vi "chkArgCompToPar.vi"(8 "error in":errorcluster, 9 "argSN":i32, 10 "arg":string, 11 "par":string) -> (0 "error out":errorcluster, 3 "judgement":string)   [LabVIEW 2010]
panel:
  out "Enum":T1(ring)=enum."float"
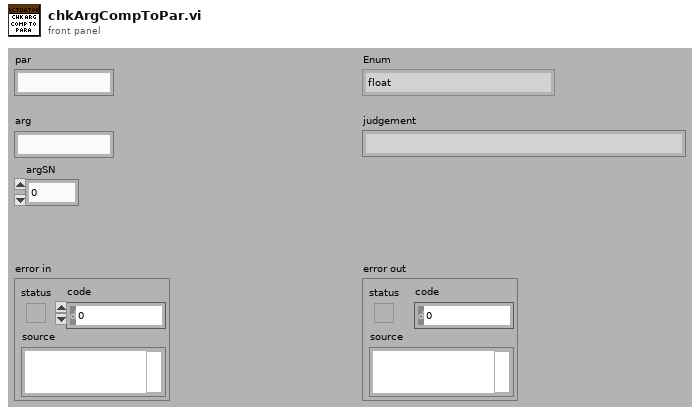
[diagram p1: front panel]
types:
  T1 = enum16{"char[]", "float", "double", "char", "int", "long", "dword", "qword", "enum"}
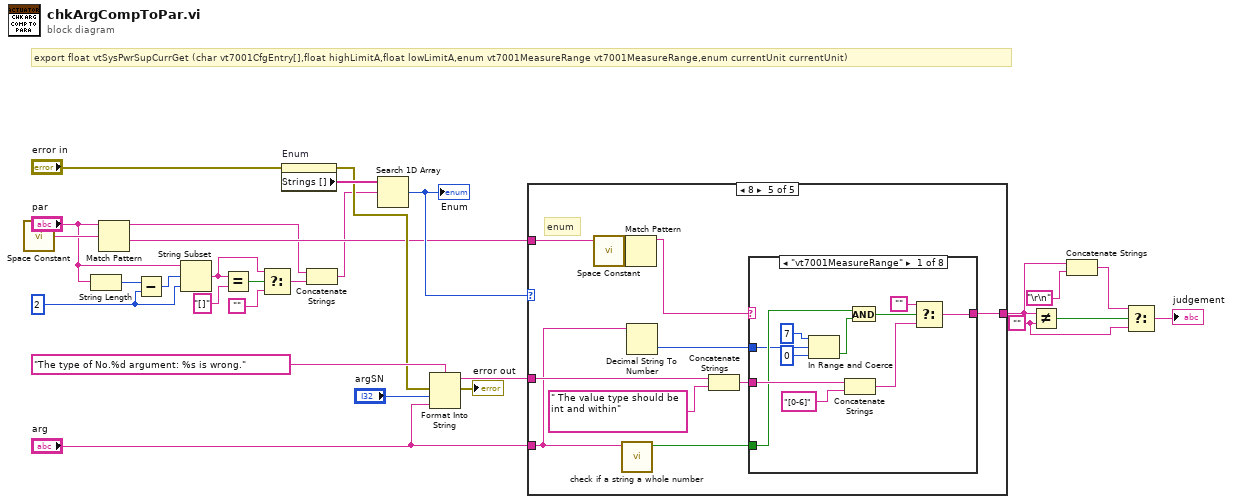
[diagram p0: block diagram]
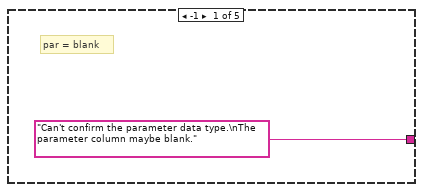
[diagram p2: hidden frame]
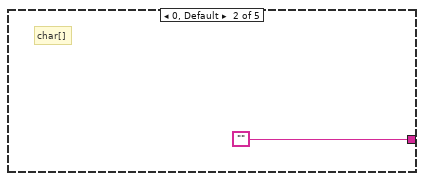
[diagram p3: hidden frame]
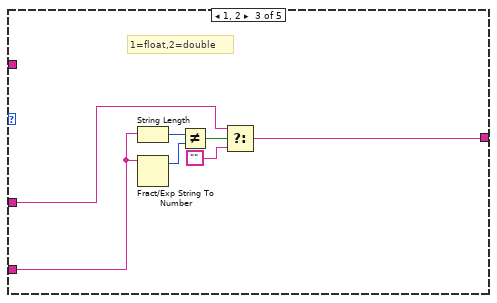
[diagram p4: hidden frame]
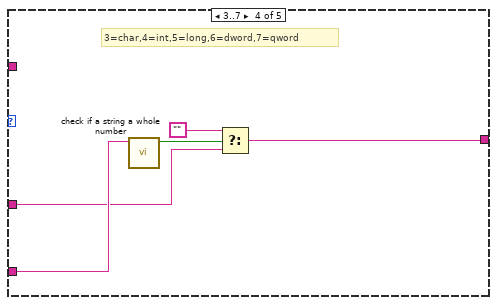
[diagram p5: hidden frame]
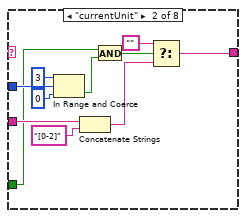
[diagram p6: hidden frame]
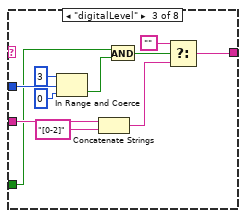
[diagram p7: hidden frame]
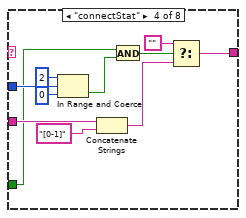
[diagram p8: hidden frame]
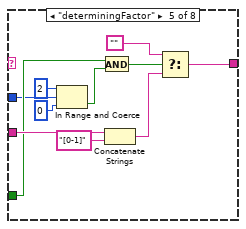
[diagram p9: hidden frame]
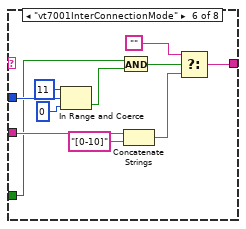
[diagram p10: hidden frame]
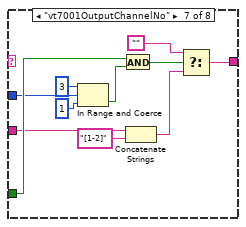
[diagram p11: hidden frame]
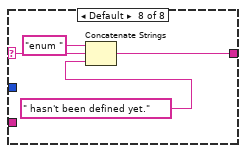
[diagram p12: hidden frame]
diagram:
  w2 = ""
  w14 = 2 ("y")
  # "export float vtSysPwrSupCurrGet (char vt7001CfgEntry[],float highLimitA,float lowLimitA,enum vt7001MeasureRange vt7001MeasureRange,enum currentUnit currentUnit)"
  n1 = call <vilib>:"Space Constant.vi"() -> ("String"=w28:string)
  n2 = String Length(string="par") -> (length=w17:i32)
  n3 = Match Pattern(string="par", regular expression=w28) -> (before substring=w8:string, after substring=w22:string)  [unwired: 1 in, 2 out]
  n4 = Subtract(x=w17, y=w14) -> (x-y=w15:i32)
  n5 = String Subset(string="par", offset (0)=w15, length (rest)=w14) -> (substring=w11:string)
  n6 = Equal?(x=w11, y="[]" ("String")) -> (x = y?=w12:bool)
  n7 = Select(t=w11, s=w12, f="") -> (s? t:f=w9:string)
  n8 = property on="Enum" class="Enum (strict)"(error in="error in") -> (error out=w24:errorcluster, "Strings []"=w27:string[])  [unwired: 1 in, 1 out]
  n9 = Concatenate Strings(w8, w9) -> (w7:string)
  n10 = Search 1D Array(1D array=w27, element=w7) -> (index of element=w26:i32)  [unwired: 1 in]
  "Enum" <- w26
  n11 = Format Into String(format string="The type of No.%d argument: %s is wrong.", error in=w24, "argSN", "arg") -> (resulting string=w23:string, error out=→"error out":errorcluster)  [unwired: 1 in]
  n12 = case shown="8" w26 {
    tunnel: "arg" -> [_ _ w35 w41 w45]
    tunnel: w23 -> [_ _ w31 w38 w47]
    tunnel: ["Can't confirm the parameter data type.\nThe parameter column maybe blank." "" w32 w42 w49] -> w4
    tunnel: w22 -> [_ _ _ _ w52]
    frame -1 {
      # "par = blank"
    }
    frame 0, Default {
      # "char[]"
    }
    frame 1, 2 {
      # "1=float,2=double"
      n13 = String Length(string=w35) -> (length=w37:i32)
      n14 = Fract/Exp String To Number(string=w35) -> (offset past number=w36:i32)  [unwired: 3 in, 1 out]
      n15 = Not Equal?(x=w37, y=w36) -> (x != y?=w34:bool)
      n16 = Select(t=w31, s=w34, f="") -> (s? t:f=w32:string)
    }
    frame 3..7 {
      # "3=char,4=int,5=long,6=dword,7=qword"
      n17 = call "check if a string a whole number.vi"("input string"=w41) -> ("is a whole number?"=w40:bool)  [unwired: 10 in]
      n18 = Select(t="", s=w40, f=w38) -> (s? t:f=w42:string)
    }
    frame 8 {
      # "enum"
      n19 = call <vilib>:"Space Constant.vi"() -> ("String"=w51:string)
      n20 = call "check if a string a whole number.vi"("input string"=w45) -> ("is a whole number?"=w48:bool)  [unwired: 10 in]
      n21 = Match Pattern(string=w52, regular expression=w51) -> (before substring=w50:string)  [unwired: 1 in, 3 out]
      n22 = Decimal String To Number(string=w45) -> (number=w44:i32)  [unwired: 2 in, 1 out]
      n23 = Concatenate Strings(w47, " The value type should be int and within" ("string")) -> (w46:string)
      n24 = case shown="\"vt7001MeasureRange\"" w50 {
        selector: w50 -> [_ _ _ _ _ _ _ w133]
        tunnel: w46 -> [w56 w67 w78 w89 w100 w110 w120 _]
        tunnel: [w55 w66 w77 w88 w101 w108 w119 w131] -> w49
        tunnel: w48 -> [w54 w64 w75 w86 w98 w109 w122 _]
        tunnel: w44 -> [w53 w65 w76 w87 w97 w111 w121 _]
        frame "vt7001MeasureRange" {
          n25 = In Range and Coerce(upper limit=7, x=w53, lower limit=0) -> (In Range?=w61:bool)  [unwired: 1 out]
          n26 = Concatenate Strings(w56, "[0-6]" ("string")) -> (w58:string)
          n27 = And(x=w54, y=w61) -> (x .and. y?=w60:bool)
          n28 = Select(t="", s=w60, f=w58) -> (s? t:f=w55:string)
        }
        frame "currentUnit" {
          n29 = In Range and Coerce(upper limit=3, x=w65, lower limit=0) -> (In Range?=w72:bool)  [unwired: 1 out]
          n30 = Concatenate Strings(w67, "[0-2]" ("string")) -> (w69:string)
          n31 = And(x=w64, y=w72) -> (x .and. y?=w71:bool)
          n32 = Select(t="", s=w71, f=w69) -> (s? t:f=w66:string)
        }
        frame "digitalLevel" {
          n33 = In Range and Coerce(upper limit=3, x=w76, lower limit=0) -> (In Range?=w83:bool)  [unwired: 1 out]
          n34 = Concatenate Strings(w78, "[0-2]" ("string")) -> (w80:string)
          n35 = And(x=w75, y=w83) -> (x .and. y?=w82:bool)
          n36 = Select(t="", s=w82, f=w80) -> (s? t:f=w77:string)
        }
        frame "connectStat" {
          n37 = In Range and Coerce(upper limit=2, x=w87, lower limit=0) -> (In Range?=w94:bool)  [unwired: 1 out]
          n38 = Concatenate Strings(w89, "[0-1]" ("string")) -> (w91:string)
          n39 = And(x=w86, y=w94) -> (x .and. y?=w93:bool)
          n40 = Select(t="", s=w93, f=w91) -> (s? t:f=w88:string)
        }
        frame "determiningFactor" {
          n41 = In Range and Coerce(upper limit=2, x=w97, lower limit=0) -> (In Range?=w105:bool)  [unwired: 1 out]
          n42 = And(x=w98, y=w105) -> (x .and. y?=w104:bool)
          n43 = Concatenate Strings(w100, "[0-1]" ("string")) -> (w99:string)
          n44 = Select(t="", s=w104, f=w99) -> (s? t:f=w101:string)
        }
        frame "vt7001InterConnectionMode" {
          n45 = In Range and Coerce(upper limit=11, x=w111, lower limit=0) -> (In Range?=w116:bool)  [unwired: 1 out]
          n46 = And(x=w109, y=w116) -> (x .and. y?=w115:bool)
          n47 = Concatenate Strings(w110, "[0-10]" ("string")) -> (w112:string)
          n48 = Select(t="", s=w115, f=w112) -> (s? t:f=w108:string)
        }
        frame "vt7001OutputChannelNo" {
          n49 = In Range and Coerce(upper limit=3, x=w121, lower limit=1) -> (In Range?=w127:bool)  [unwired: 1 out]
          n50 = And(x=w122, y=w127) -> (x .and. y?=w126:bool)
          n51 = Concatenate Strings(w120, "[1-2]" ("string")) -> (w123:string)
          n52 = Select(t="", s=w126, f=w123) -> (s? t:f=w119:string)
        }
        frame Default {
          n53 = Concatenate Strings("enum " ("string"), w133, " hasn't been defined yet.") -> (w131:string)
        }
      }
    }
  }
  n54 = Not Equal?(x=w4, y=w2) -> (x != y?=w6:bool)
  n55 = Concatenate Strings(w4, "\r\n") -> (w3:string)
  n56 = Select(t=w3, s=w6, f=w2) -> (s? t:f=→"judgement":string)
